vi "Read Temperature F.vi"(7 "Use Cached Data?":bool, 8 "Error In":errorcluster, 10 "Device Name":string, 11 "Nest Config":T1) -> (0 "Error Out":errorcluster, 2 "Current Temp (F)":dbl, 3 "Nest Config":T1)   [LabVIEW 2013, in "LVH-Nest.lvlib"]
doc: "Read current temperatuer in Fahrenheit."
uses:
  LVH-Nest.lvlib
  Private/Type Defs/Nest Config.ctl
  <vilib>/httpClient/ClientHandle.ctl
  Private/Type Defs/Session Data.ctl
  <vilib>/httpClient/LabVIEWHTTPClient.lvlib
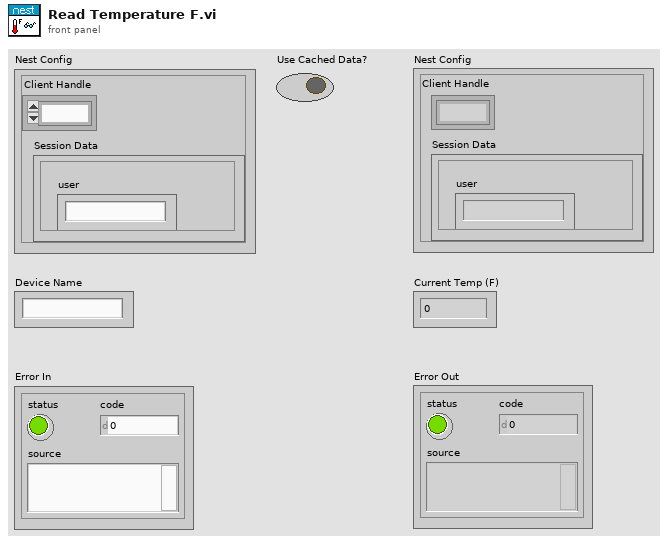
[diagram p1: front panel]
types:
  T1 = typedef "LVH-Nest.lvlib/Nest Config.ctl" = cluster{"Client Handle":T2, "Session Data":T3}
  T2 = typedef "LabVIEWHTTPClient.lvlib/ClientHandle.ctl" = refnum<k1>
  T3 = typedef "LVH-Nest.lvlib/Session Data.ctl" = cluster{"is_superuser":bool, "is_staff":bool, "urls":cluster{"transport_url":string, "rubyapi_url":string, "weather_url":string, "log_upload_url":string, "support_url":string}, "limits":cluster{"thermostats_per_structure":u32, "structures":u32, "thermostats":u32, "smoke_detectors":u32, "smoke_detectors_per_structure":u32}, "access_token":string, "userid":string, "expires_in":string, "email":string, "user":string, "language":string}
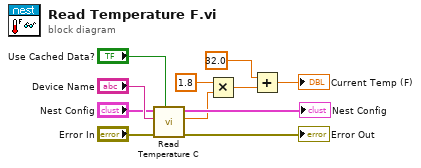
[diagram p0: block diagram]
diagram:
  n1 = call "Read Temperature C.vi"("Use Cached Data?"="Use Cached Data?", "Error In"="Error In", "Device Name"="Device Name", "Nest Config"="Nest Config") -> ("Error Out"=→"Error Out":errorcluster, "Current Temp (C)"=w2:dbl, "Nest Config"=→"Nest Config":T1)  [unwired: 5 in]
  n2 = Multiply(x=1.8 ("y"), y=w2) -> (x*y=w4:dbl)
  n3 = Add(x=32.0, y=w4) -> (x+y=→"Current Temp (F)":dbl)
